vi "Stop.vi"(8 "error in (no error)":errorcluster, 11 "Pub Sub Message Channel in":refnum<class "Pub Sub Message Channel.lvclass">) -> (0 "error out":errorcluster, 3 "Pub Sub Message Channel out":refnum<class "Pub Sub Message Channel.lvclass">)   [LabVIEW 2020, in "Actor Pub Sub Channels.lvlib" / "Pub Sub Message Channel.lvclass"]
uses:
  Pub Sub Message Channel.lvclass
  Close Channel Message/Close Channel Message.lvclass
  C:/Program Files (x86)/National Instruments/LabVIEW 2020/vi.lib/ActorFramework/Message/Message.lvclass
  Pub Sub Message Channel.lvclass/Pub Sub Message Channel.ctl
  <vilib>/ActorFramework/Message Queue/Message Queue.lvclass/Message Queue.ctl
  <vilib>/ActorFramework/Self-Addressed Msg/Self-Addressed Msg.lvclass/Self-Addressed Msg.ctl
  <vilib>/ActorFramework/Self-Addressed Msg/Self-Addressed Msg.lvclass
  <vilib>/ActorFramework/Message Queue/Message Queue.lvclass
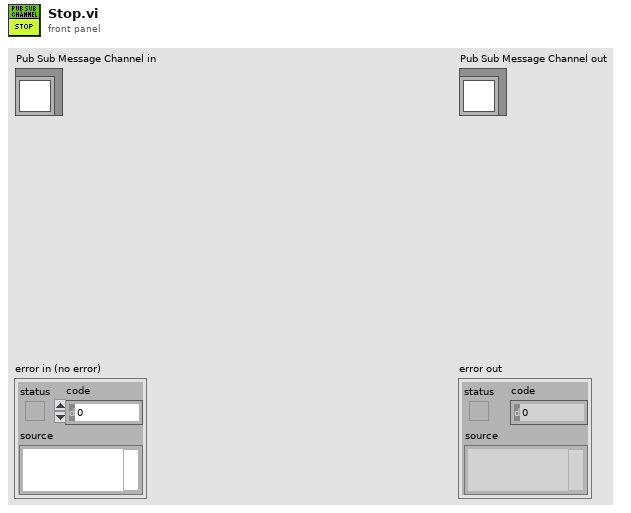
[diagram p1: front panel]
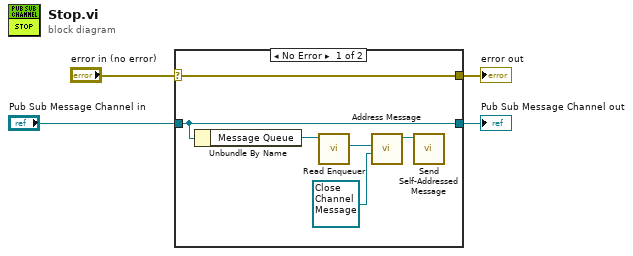
[diagram p0: block diagram]
diagram:
  n1 = case shown="No Error" "error in (no error)" {
    selector: "error in (no error)" -> [w10 w12]
    tunnel: [w10 w12] -> w3
    tunnel: [w9 w11] -> w1
    tunnel: "Pub Sub Message Channel in" -> [w9 w11]
    frame No Error {
      n2 = Unbundle By Name(w9) -> ("Message Queue"=w8:refnum<class "Message Queue.lvclass">)
      n3 = call <vilib>:"Read Enqueuer.vi"("Message Queue"=w8) -> ("Message Enqueuer"=w6:refnum<class "Message Enqueuer.lvclass">)  [unwired: 10 in]
      n4 = call <vilib>:"Address Message.vi"("Message"=refnum<class "Close Channel Message.lvclass"> refnum ("Actor Pub Sub Channels.lvlib:Close Channel Message.lvclass"), "Destination"=w6) -> ("Self-Addressed Message"=w5:refnum<class "Self-Addressed Msg.lvclass">)  [unwired: 9 in]
      n5 = call-dynamic "Send Self-Addressed Message.vi"("Self-Addressed Message in"=w5) -> ()  [unwired: 9 in, 2 out]
    }
    frame Error {
    }
  }
  "error out" <- w3
  "Pub Sub Message Channel out" <- w1
